vi "Popup with timeout.vi"(8 "error":errorcluster, 10 "timeout":u32, 11 "message":string) -> (0 "error out":errorcluster)   [LabVIEW 2013]
panel:
  in  "Boolean":bool
  out "String":string
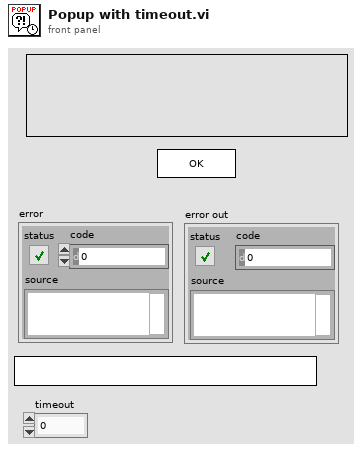
[diagram p1: front panel]
types:
  T1 = enum32{"Invalid", "Standard", "Closed", "Hidden", "Minimized", "Maximized"}
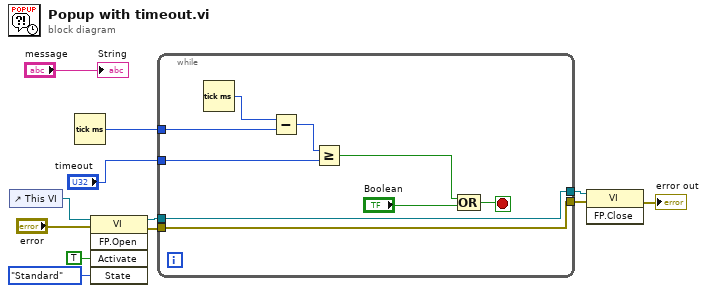
[diagram p0: block diagram]
diagram:
  n1 = control-ref of="This VI"() -> (w6:refnum<vi>)
  n2 = Tick Count (ms)() -> (millisecond timer value=w12:u32)
  n3 = invoke class="VI" method="FP.Open"(reference=w6, error in="error", "Activate"=TRUE ("Activate?"), "State"=T1."Standard") -> (reference out=w3:refnum<vi>, error out=w5:errorcluster)  [unwired: 1 in, 3 out]
  n4 = while {
    tunnel: w12 -> [w20]
    tunnel: "timeout" -> [w18]
    tunnel: [w14] -> w10
    tunnel: w5 -> [w14]
    tunnel: [w13] -> w4
    tunnel: w3 -> [w13]
    stop <- w15 stop-if-true
    n5 = Tick Count (ms)() -> (millisecond timer value=w21:u32)
    n6 = Subtract(x=w21, y=w20) -> (x-y=w19:u32)
    n7 = Greater Or Equal?(x=w19, y=w18) -> (x >= y?=w17:bool)
    n8 = Compound Arithmetic op=OR(w17, "Boolean") -> (w15:bool)
  }
  n9 = invoke class="VI" method="FP.Close"(reference=w4, error in=w10) -> (error out=→"error out":errorcluster)  [unwired: 1 in, 2 out]
  "String" <- "message"
